vi "poly conversion.vi"(10 "Volts":dbl format="%.2f", 11 "conversion matrix":sgl[][](array[numeric]) format="%.2f") -> (3 "Calibrated value":dbl format="%.2f")   [LabVIEW 2015]
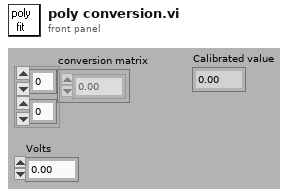
[diagram p1: front panel]
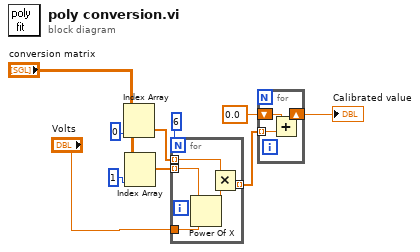
[diagram p0: block diagram]
diagram:
  n1 = Index Array(array="conversion matrix", index (col)=0) -> (element=w4:sgl[])  [unwired: 1 in]
  n2 = Index Array(array="conversion matrix", index (col)=1) -> (element=w3:sgl[])  [unwired: 1 in]
  n3 = for {
    N: 6 -> [_]
    tunnel: "Volts" -> [w15]
    tunnel: w3 -> [w14] mode=indexing
    tunnel: w4 -> [w13] mode=indexing
    tunnel: [w11] -> w1 mode=indexing
    n4 = Power Of X(1:w15, 2:w14) -> (0:w12:dbl)
    n5 = Multiply(x=w13, y=w12) -> (x*y=w11:dbl)
  }
  n6 = for {
    tunnel: w1 -> [w18] mode=indexing
    shift-right: [w16] -> w10
    shift-left: sgl 0.0 -> [w17]
    n7 = Add(x=w17, y=w18) -> (x+y=w16:dbl)
  }
  "Calibrated value" <- w10
